vi "MaxXY.vi"(1 "input_xyz_um":T2, 2 "parameters_xy_scan":T1={"image_size_xy_um"=1.0, "frame_size_xy_px"=10, "pixel_dwell_ms"=1.0} {"pixel_dwell_ms" format="%#_13g"; "image_size_xy_um" format="%#_13g"}) -> (7 "output_xyz_um":T2, 8 "BestGaussianFit":cluster{dbl[], dbl[]}, 9 "SumXY":cluster{dbl[], dbl[]}, 10 "image":dbl[][](graph))   [LabVIEW 2018]
uses:
  <vilib>/Analysis/1siggen.llb/Ramp Pattern by Samples.vi
  <vilib>/Analysis/NI_AALPro.lvlib
  <vilib>/Analysis/NI_AALBase.lvlib
panel:
  in  "gaussian_fit":bool=TRUE
  out "section_Y":dbl[][](graph)
  out "section_X":dbl[][](graph)
  in  "scan_direction":enum32{"0", "1"}(radio) caption="Scan direction:"
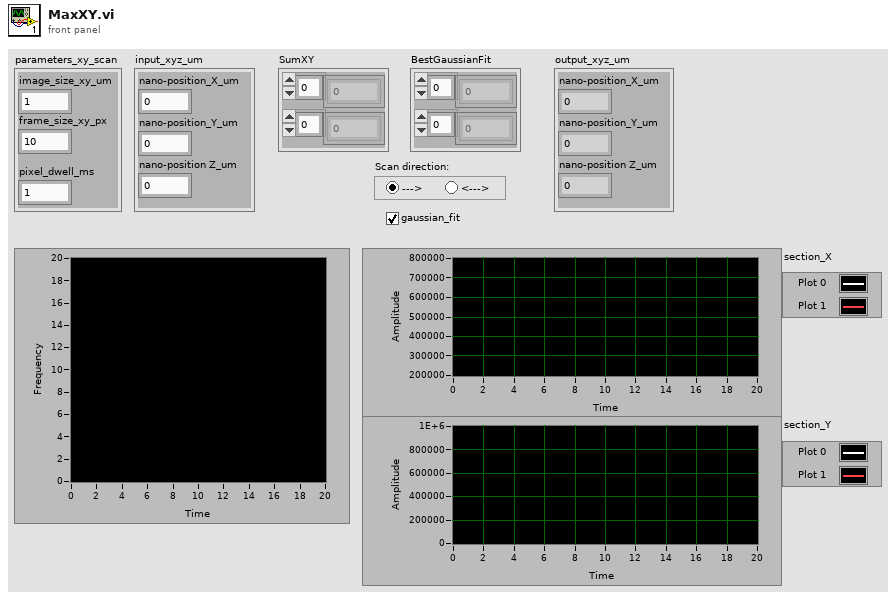
[diagram p1: front panel]
types:
  T1 = cluster{"image_size_xy_um":dbl, "frame_size_xy_px":u32, "pixel_dwell_ms":dbl}
  T2 = cluster{"nano-position_X_um":sgl, "nano-position_Y_um":sgl, "nano-position Z_um":sgl}
  T3 = cluster{"Best Gaussian Fit":dbl[], "Best Gaussian Fit":dbl[]}
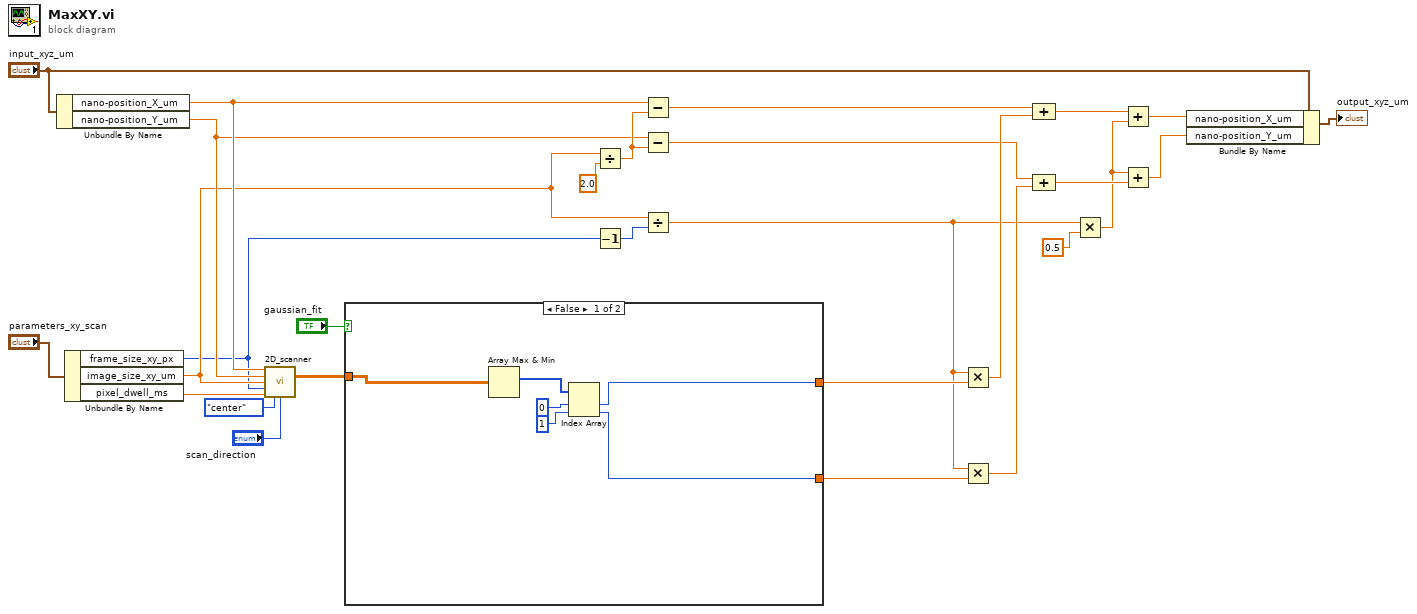
[diagram p0: block diagram]
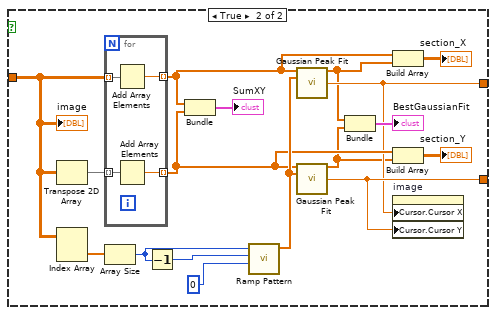
[diagram p2: hidden frame]
diagram:
  n1 = Unbundle By Name("input_xyz_um") -> ("nano-position_X_um"=w9:sgl, "nano-position_Y_um"=w8:sgl)
  n2 = Unbundle By Name("parameters_xy_scan") -> ("frame_size_xy_px"=w6:u32, "image_size_xy_um"=w7:dbl, "pixel_dwell_ms"=w5:dbl)
  n3 = call "2D_scanner.vi"("pos-start_x"=w9, "pos-start_y"=w8, "image_size_x_um"=w7, "frame_size_x_px"=w6, "pixel_dwell_ms"=w5, "pos_start"=enum32{"bottom-left", "center"}."center", "scan_direction"="scan_direction") -> ("image_out"=w2:dbl[][])  [unwired: 8 in]
  n4 = case shown="False" "gaussian_fit" {
    tunnel: [w31 w39] -> w21
    tunnel: [w32 w38] -> w20
    tunnel: w2 -> [w29 w35]
    frame False {
      n5 = Array Max & Min(array=w29) -> (max index (indices)=w33:i32[])  [unwired: 3 out]
      n6 = Index Array(array=w33, index #1=0 ("index"), index #2=1 ("index")) -> (element #1=w32:i32, element #2=w31:i32)
    }
    frame True {
      n7 = Transpose 2D Array(2D array=w35) -> (transposed array=w51:dbl[][])
      n8 = Index Array(array=w35) -> (element=w50:dbl[])  [unwired: 2 in]
      n9 = for {
        tunnel: w35 -> [w55] mode=indexing
        tunnel: w51 -> [w54] mode=indexing
        tunnel: [w53] -> w40 mode=indexing
        tunnel: [w52] -> w42 mode=indexing
        n10 = Add Array Elements(numeric array=w55) -> (sum=w53:dbl)
        n11 = Add Array Elements(numeric array=w54) -> (sum=w52:dbl)
      }
      n12 = Array Size(array=w50) -> (size(s)=w49:i32)
      n13 = Decrement(x=w49) -> (x-1=w48:i32)
      n14 = Bundle(w40, w42) -> (→"SumXY":cluster{dbl[], dbl[]})  [unwired: 1 in]
      n15 = call-poly <vilib>:"Ramp Pattern.vi"("start"=u32 0, "end"=w48, "samples"=w49) -> ("Ramp Pattern"=w46:dbl[])  [unwired: 7 in, 1 out]
      n16 = call <vilib>:"Gaussian Peak Fit.vi"("Y"=w40, "X"=w46) -> ("Best Gaussian Fit"=w37:dbl[], "center"=w38:dbl)  [unwired: 7 in, 5 out]
      n17 = call <vilib>:"Gaussian Peak Fit.vi"("Y"=w42, "X"=w46) -> ("Best Gaussian Fit"=w36:dbl[], "center"=w39:dbl)  [unwired: 7 in, 5 out]
      n18 = Bundle("Best Gaussian Fit"=w37, "Best Gaussian Fit"=w36) -> (→"BestGaussianFit":T3)  [unwired: 1 in]
      n19 = Build Array(w40, w37) -> (→"section_X":dbl[][])
      n20 = Build Array(w42, w36) -> (→"section_Y":dbl[][])
      n21 = property on="image" class="IntGraph (strict)"("Cursor.Cursor X"=w38, "Cursor.Cursor Y"=w39) -> ()  [unwired: 2 in, 2 out]
      "image" <- w35
    }
  }
  n22 = Divide(x=w7, y=2.0) -> (x/y=w24:dbl)
  n23 = Decrement(x=w6) -> (x-1=w22:u32)
  n24 = Subtract(x=w9, y=w24) -> (x-y=w23:dbl)
  n25 = Subtract(x=w8, y=w24) -> (x-y=w13:dbl)
  n26 = Divide(x=w7, y=w22) -> (x/y=w19:dbl)
  n27 = Multiply(x=w19, y=w20) -> (x*y=w26:dbl)
  n28 = Multiply(x=w19, y=w21) -> (x*y=w28:dbl)
  n29 = Compound Arithmetic op=ADD(w23, w26) -> (w16:dbl)
  n30 = Compound Arithmetic op=ADD(w13, w28) -> (w27:dbl)
  n31 = Multiply(x=w19, y=0.5) -> (x*y=w17:dbl)
  n32 = Add(x=w16, y=w17) -> (x+y=w12:dbl)
  n33 = Add(x=w17, y=w27) -> (x+y=w11:dbl)
  n34 = Bundle By Name(cluster="input_xyz_um", "nano-position_X_um"=w12, "nano-position_Y_um"=w11) -> (→"output_xyz_um":T2)
